vi "NanoBright Acquisition preview source code.vi"(2 "Acquisition\nTime (s)":u32=10, 3 "Acquisition Rate (Hz)":dbl=1000.0 caption="Acquisition\nRate (Hz)") -> ()   [LabVIEW 2014]
uses:
  C:/Program Files (x86)/National Instruments/LabVIEW 2014/vi.lib/ULx/ULx_LV.dll
  Program Files (x86)/National Instruments/LabVIEW 2014/vi.lib/ULx/ULx_LV.dll
  <vilib>/Utility/error.llb/DialogType.ctl
  <vilib>/Analysis/baseanly.llb/Mean (DBL).vi
  <vilib>/ULx/Create Channel.llb/ULx Create Channel (CI-Count Edges).vi
  <vilib>/ULx/Timing.llb/ULx Timing (Sample Clock).vi
  <vilib>/ULx/Read.llb/ULx Read (Counter 2D U32 NChan NSamp).vi
  <vilib>/Analysis/NI_AALBase.lvlib
panel:
  out "Buffer":dbl=100.0
  out "Samples/loop":i32=10
  out "Channel 1":dbl format="%#_3g"
  out "Channel 2":dbl format="%#_3g"
  out "Signal":u32[][](graph)
  in  "Clock Source":i32(ring) items=["OnboardClock", "ExternalClock", "NoClock"]
  in  "Count Direction":i32(ring) items=["CountUp", "CountDown"]
  in  "Edge":i32(ring) items=["Rising", "Falling"]
  in  "Counter(s)":refnum<k21>="Dev0/Ci0:1"
  in  "Initial Count":u32
  in  "stop":bool
  # "Signal Averages"
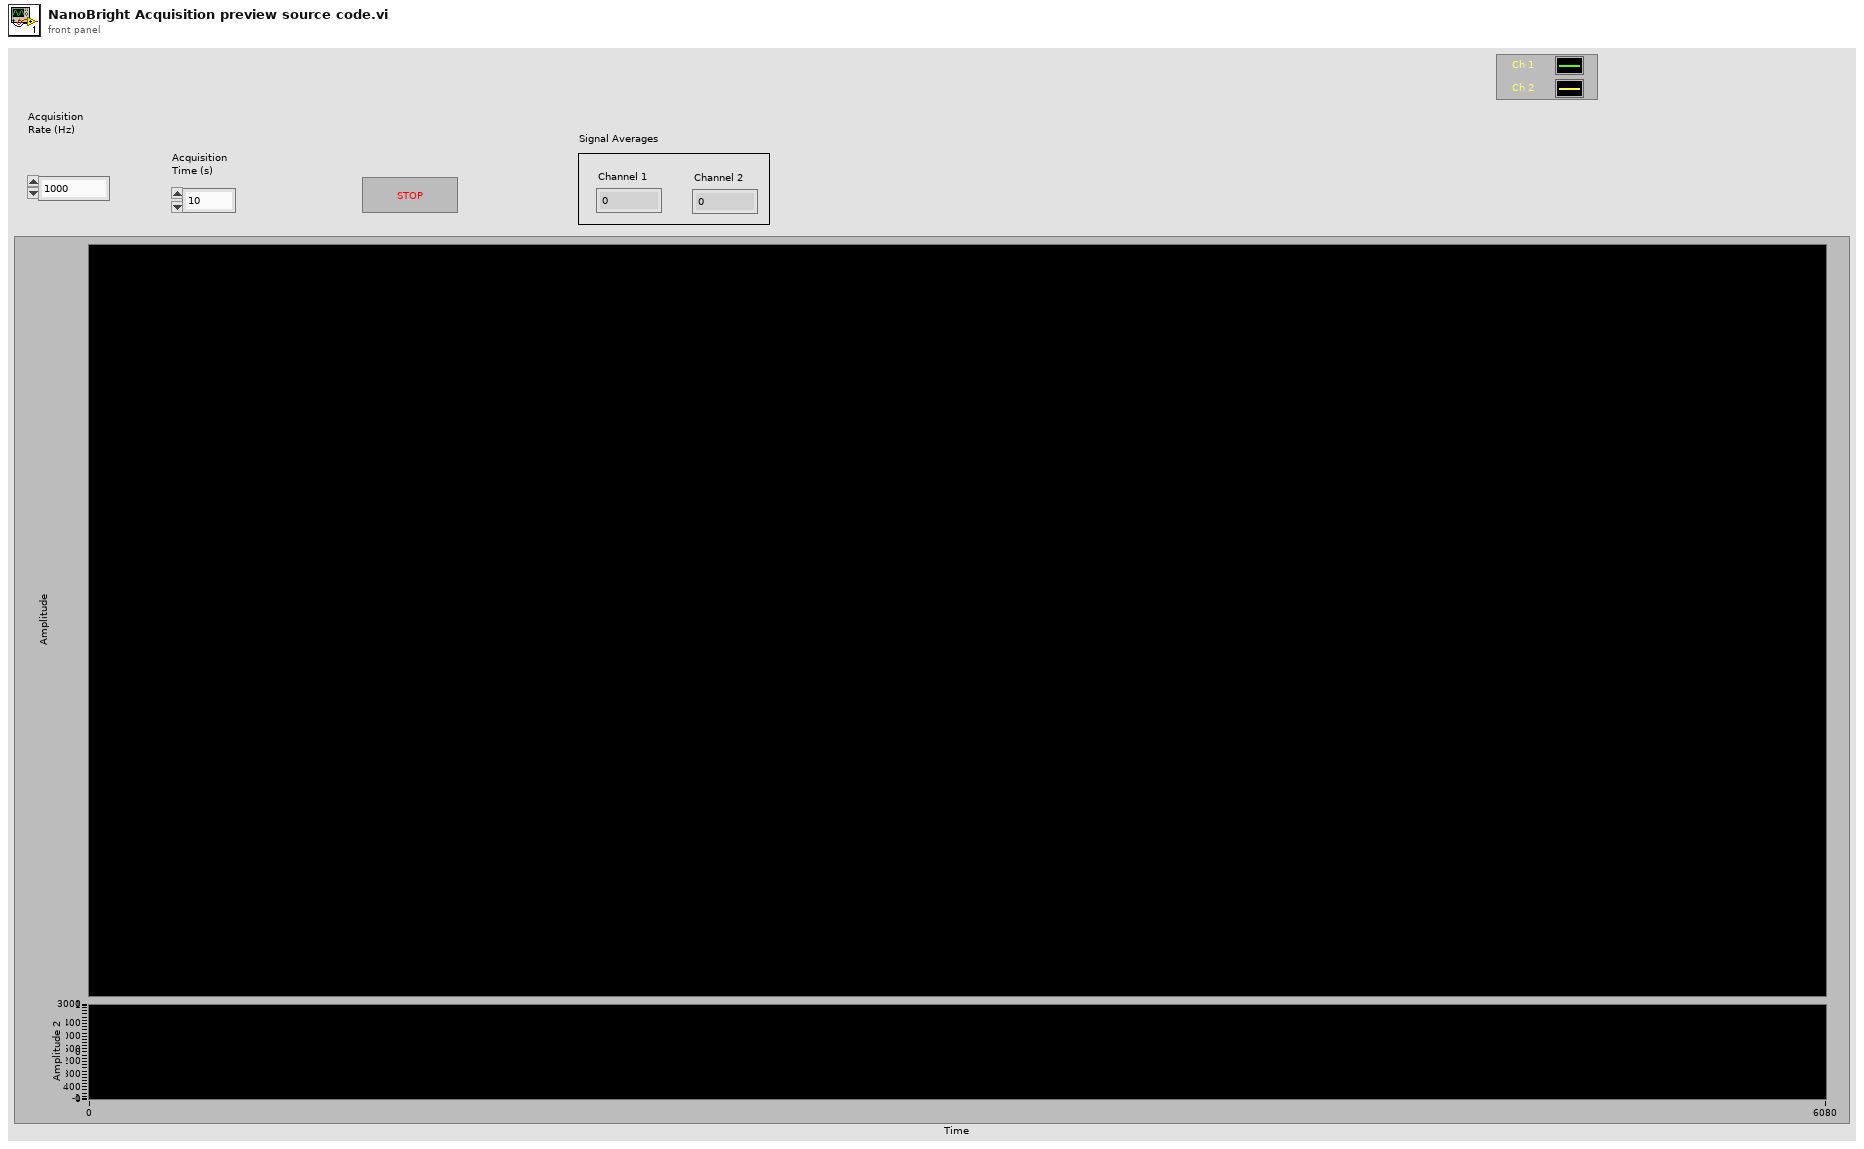
[diagram p1: front panel]
types:
  T1 = typedef "DialogType.ctl" = u16
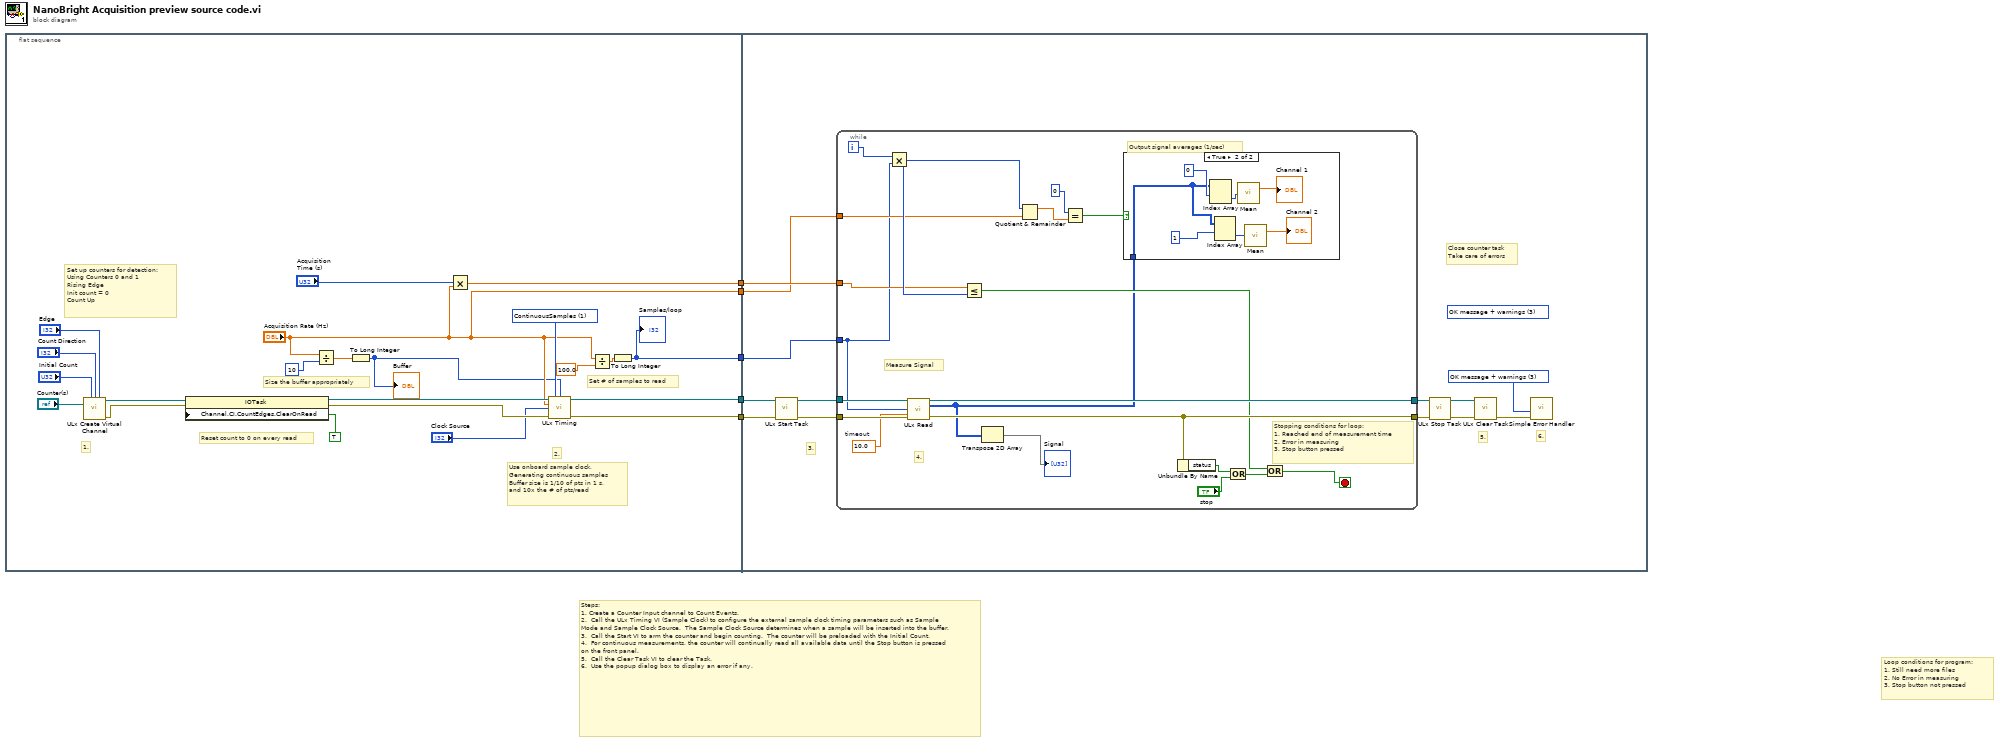
[diagram p0: block diagram]
diagram:
  # "Loop conditions for program:\n1. Still need more files\n2. No Error in measuring\n3. Stop button not pressed"
  # "Steps: \n1. Create a Counter Input channel to Count Events.\n2.  Call the ULx Timing VI (Sample Clock) to configure the external sample clock timing parameters such as Sample Mode and Sample Clock Source.  The Sample Clock Source determines when a sample will be inserted into the buffer.\n3.  Call the Start VI to arm the counter and begin counting.  The counter will be preloaded with the Initial Count.\n4.  For continuous measurements, the counter will continually read all available data until the Stop button is pressed on the front panel.\n5.  Call the Clear Task VI to clear the Task.\n6.  Use the popup dialog box to display an error if any."
  n1 = flat-sequence {
    tunnel: [w17] -> w5
    tunnel: [w15] -> w4
    tunnel: [w16] -> w3
    tunnel: ["Acquisition Rate (Hz)"] -> w2
    tunnel: [w7] -> w1
    tunnel: w5 -> [w32]
    tunnel: w4 -> [w31]
    tunnel: w3 -> [w30]
    tunnel: w2 -> [w29]
    tunnel: w1 -> [w28]
    frame #0 {
      w18 = 1 items=["FiniteSamples", "ContinuousSamples"] ("sample mode")
      # "Use onboard sample clock,\nGenerating continuous samples\nBuffer size is 1/10 of pts in 1 s, \nand 10x the # of pts/read"
      # "Reset count to 0 on every read"
      # "Set up counters for detection:\nUsing Counters 0 and 1\nRising Edge\nInit count = 0\nCount Up"
      # "Set # of samples to read"
      # "Size the buffer appropriately"
      # "2."
      # "1."
      n2 = call-poly <vilib>:"ULx Create Virtual Channel.vi"("initial count"="Initial Count", "count direction"="Count Direction", "edge"="Edge", "counters"="Counter(s)") -> ("task out"=w14:refnum<k24>, "error out"=w13:errorcluster)  [unwired: 10 in]
      n3 = property class="IOTask"(reference=w14, error in=w13, "Channel.CI.CountEdges.ClearOnRead"=TRUE) -> (reference out=w25:refnum<k24>, error out=w26:errorcluster)
      n4 = Divide(x="Acquisition Rate (Hz)", y=10 ("samples per channel")) -> (x/y=w11:dbl)
      n5 = To Long Integer(number=w11) -> (32bit integer=w6:i32)
      "Buffer" <- w6
      n6 = Multiply(x="Acquisition\nTime (s)", y="Acquisition Rate (Hz)") -> (x*y=w17:dbl)
      n7 = call-poly <vilib>:"ULx Timing.vi"("task in"=w25, "sample mode"=w18, "samples per channel"=w6, "rate"="Acquisition Rate (Hz)", "clock source"="Clock Source", "error in"=w26) -> ("task out"=w16:refnum<k24>, "error out"=w15:errorcluster)  [unwired: 8 in]
      n8 = Divide(x="Acquisition Rate (Hz)", y=100.0) -> (x/y=w8:dbl)
      n9 = To Long Integer(number=w8) -> (32bit integer=w7:i32)
      "Samples/loop" <- w7
    }
    frame #1 {
      (unwired) T1 3 items=["no dialog", "OK message", "continue or stop message", "OK message + warnings", "continue/stop + warnings"] ("type of dialog (OK msg:1)")
      w37 = T1 3 items=["no dialog", "OK message", "continue or stop message", "OK message + warnings", "continue/stop + warnings"] ("type of dialog (OK msg:1)")
      # "Close counter task\nTake care of errors"
      # "6."
      # "5."
      # "3."
      n10 = call <vilib>:"ULx Start Task.vi"("task in"=w30, "error in"=w31) -> ("task out"=w38:refnum<k24>, "error out"=w40:errorcluster)  [unwired: 12 in]
      n11 = while {
        tunnel: w40 -> [w60]
        tunnel: [w54] -> w35
        tunnel: w38 -> [w57]
        tunnel: [w55] -> w36
        tunnel: w32 -> [w48]
        tunnel: w29 -> [w45]
        tunnel: w28 -> [w44]
        i -> [w43]
        stop <- w47 stop-if-true
        w56 = 10.0  # timeout
        # "Output signal averages (1/sec)"
        # "Stopping conditions for loop:\n1. Reached end of measurement time\n2. Error in measuring\n3. Stop button pressed"
        # "Measure Signal"
        # "4."
        n12 = Multiply(x=w43, y=w44) -> (x*y=w52:i32)
        n13 = call-poly <vilib>:"ULx Read.vi"("task in"=w57, "number of samples per channel"=w44, "timeout"=w56, "error in"=w60) -> ("task out"=w55:refnum<k24>, "data"=w41:u32[][], "error out"=w54:errorcluster)  [unwired: 9 in]
        n14 = Less Or Equal?(x=w48, y=w52) -> (x <= y?=w53:bool)
        n15 = Transpose 2D Array(2D array=w41) -> (transposed array=→"Signal":u32[][])
        n16 = Quotient & Remainder(x=w52, y=w45) -> (x-y*floor(x/y)=w51:dbl)  [unwired: 1 out]
        n17 = Equal?(x=0, y=w51) -> (x = y?=w49:bool)
        n18 = case shown="True" w49 {
          tunnel: w41 -> [_ w61]
          frame False {
          }
          frame True {
            n19 = Index Array(array=w61, index (row)=0) -> (element=w65:u32[])  [unwired: 1 in]
            n20 = Index Array(array=w61, index (row)=1) -> (element=w64:u32[])  [unwired: 1 in]
            n21 = call-poly <vilib>:"Mean.vi"("X"=w65) -> ("mean"=→"Channel 1":dbl)  [unwired: 1 out]
            n22 = call-poly <vilib>:"Mean.vi"("X"=w64) -> ("mean"=→"Channel 2":dbl)  [unwired: 1 out]
          }
        }
        n23 = Unbundle By Name(w54) -> ("status"=w58:bool)
        n24 = Or(x=w58, y="stop") -> (x .or. y?=w46:bool)
        n25 = Or(x=w53, y=w46) -> (x .or. y?=w47:bool)
      }
      n26 = call <vilib>:"ULx Stop Task.vi"("error in"=w35, "task in"=w36) -> ("error out"=w33:errorcluster, "task out"=w34:refnum<k24>)  [unwired: 8 in]
      n27 = call <vilib>:"ULx Clear Task.vi"("task in"=w34, "error in"=w33) -> ("error out"=w39:errorcluster)  [unwired: 13 in]
      n28 = call <vilib>:"Simple Error Handler.vi"("type of dialog (OK msg:1)"=w37, "error in (no error)"=w39) -> ()  [unwired: 3 in, 5 out]
    }
  }
